vi "XBox Control Launcher.vi"() -> (0 "XBox Event Ref":T1)   [LabVIEW 2015]
uses:
  XBox-Events Ref.ctl
  XBox-Globals.vi
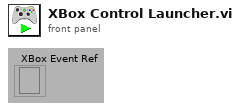
[diagram p1: front panel]
types:
  T1 = typedef "XBox-Events Ref.ctl" = refnum<event-registration>
  T2 = enum32{"Invalid", "Standard", "Closed", "Hidden", "Minimized", "Maximized"}
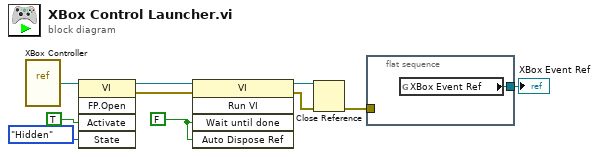
[diagram p0: block diagram]
diagram:
  w1 = FALSE ("Wait Until Done")
  n1 = vi-ref "XBox Controller.vi"() -> (w7:refnum<vi>)
  n2 = invoke class="VI" method="FP.Open"(reference=w7, "Activate"=TRUE ("Activate?"), "State"=T2."Hidden") -> (reference out=w4:refnum<vi>, error out=w5:errorcluster)  [unwired: 2 in, 3 out]
  n3 = invoke class="VI" method="Run VI"(reference=w4, error in=w5, "Wait until done"=w1, "Auto Dispose Ref"=w1) -> (reference out=w6:refnum<vi>, error out=w8:errorcluster)  [unwired: 1 in, 3 out]
  n4 = Close Reference(reference=w6, error in (no error)=w8) -> (error out=w10:errorcluster)
  n5 = flat-sequence {
    tunnel: [w11] -> w9
    tunnel: w10 -> [_]
    frame #0 {
      n6 = global read "XBox-Globals.vi" "XBox Event Ref"() -> (w11:T1)
    }
  }
  "XBox Event Ref" <- w9
